vi "Destroy.vi"(8 "Error In":errorcluster, 11 "Reader":refnum<class "Reader.lvclass">) -> (0 "Error Out":errorcluster)   [LabVIEW 2018, in "Toolkit.lvlib" / "Reader.lvclass"]
doc: "Destroys an object of the Reader class. This must be called when shutting down an application to avoid memory leaks. This may free resources."
uses:
  Reader.lvclass
  Reader.lvclass/Reader.ctl
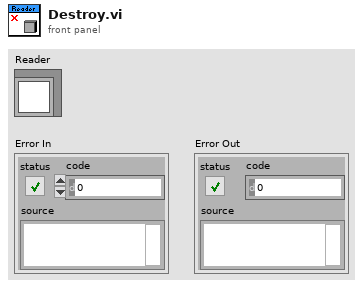
[diagram p1: front panel]
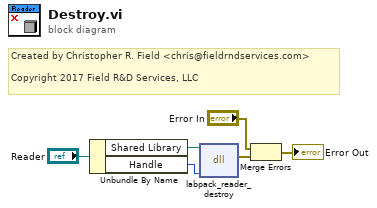
[diagram p0: block diagram]
diagram:
  # "Created by Christopher R. Field <chris@fieldrndservices.com>\n\nCopyright 2017 Field R&D Services, LLC"
  n1 = Unbundle By Name("Reader") -> ("Shared Library"=w5:path, "Handle"=w4:u64)
  n2 = dll-call lib="D:/Users/cfield/Code/MessagePack/LabPack/LabVIEW/trunk/src/LabPack/Private/labpack-x64.dll" fn="labpack_reader_destroy"(path in=w5, "reader"=w4) -> (error out=w3:errorcluster)  [unwired: 4 in, 1 out]
  n3 = Merge Errors("Error In", w3) -> (→"Error Out":errorcluster)
